vi "demo.vi"() -> ()   [LabVIEW 2019]
panel:
  out "输出数组":u16[][](array[numeric])
  out "buf":u16[](array[numeric])
  out "Image":T1(plugin-control)
  in  "停止":bool
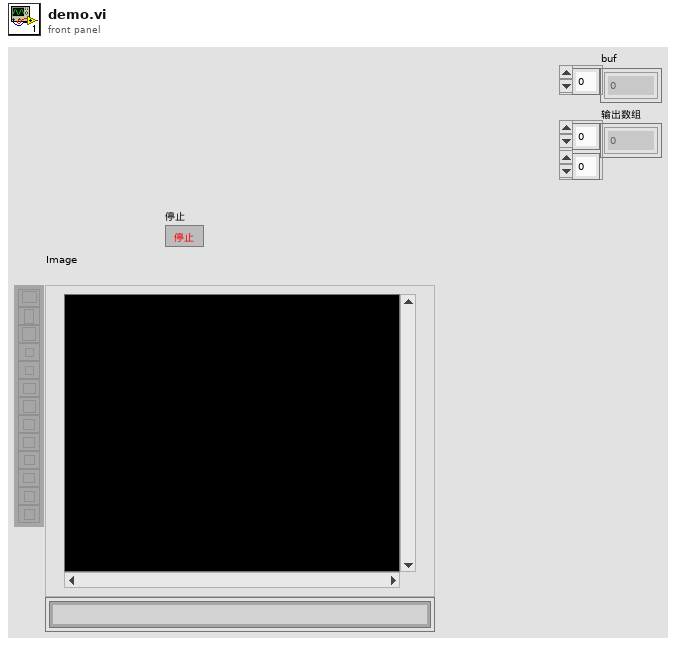
[diagram p1: front panel]
types:
  T1 = typedef "IMAQ Image.ctl" = refnum<image>
  T2 = typedef "Image Type" = u32
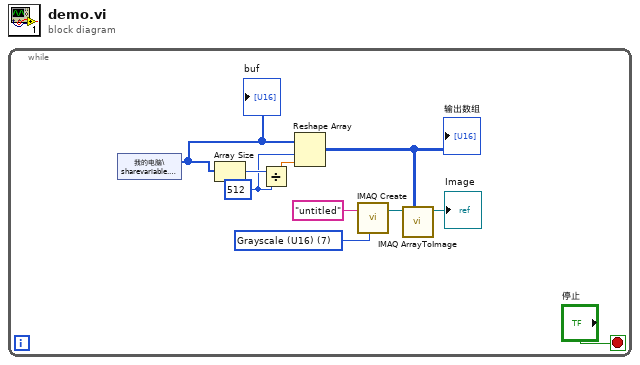
[diagram p0: block diagram]
diagram:
  n1 = while {
    stop <- "停止" stop-if-true
    w2 = 512 ("y")
    w6 = T2 7 items=["Grayscale (U8)", "Grayscale (I16)", "Grayscale (SGL)", "Complex (CSG)", "RGB (U32)", "HSL (U32)", "RGB (U64)", "Grayscale (U16)"] ("Image Type")
    n2 = shared-variable "我的电脑\\sharevariable.lvlib\\buf"() -> (w5:u16[])  [unwired: 1 in, 1 out]
    "buf" <- w5
    n3 = Array Size(array=w5) -> (size(s)=w4:i32)
    n4 = Divide(x=w4, y=w2) -> (x/y=w3:dbl)
    n5 = Reshape Array(w5, w2, w3) -> (w1:u16[][])
    "输出数组" <- w1
    n6 = call "IMAQ Create"("Image Name"="untitled", "Image Type"=w6) -> ("New Image"=w9:T1)  [unwired: 3 in, 1 out]
    n7 = call "IMAQ ArrayToImage"("Image Pixels (U16)"=w1, "Image"=w9) -> ("Image Out"=→"Image":T1)  [unwired: 8 in, 1 out]
  }
